vi "Symphony Init.vi"(0 "Device Names":refnum<vi>, 1 "Device IDs":refnum<vi>) -> ()   [LabVIEW 2010]
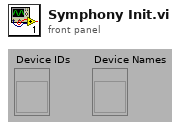
[diagram p1: front panel]
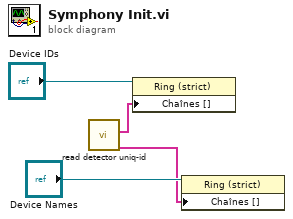
[diagram p0: block diagram]
diagram:
  n1 = call "read detector uniq-id.vi"() -> ("UniqueID"=w1:string[], "Name"=w2:string[])  [unwired: 5 out]
  n2 = property on="Property Node" class="Ring (strict)"(reference="Device IDs", "Chaînes []"=w1) -> ()  [unwired: 1 in, 2 out]
  n3 = property on="Property Node" class="Ring (strict)"(reference="Device Names", "Chaînes []"=w2) -> ()  [unwired: 1 in, 2 out]
